vi "Set Color.vi"(9 "index":i32, 10 "Flat Legend":cluster{"Color Box":u32, "String":string}[](array[cluster]), 11 "list in":T1[](array[typedef]) {"Creation Date" format="%<%x>T"; "Last Updated" format="%<%x>T"}) -> (3 "list out":T1[](array[typedef]) {"Creation Date" format="%<%x>T"; "Last Updated" format="%<%x>T"})   [LabVIEW 2018]
uses:
  Type Defs/SR Cluster.ctl
  Type Defs/SR Status.ctl
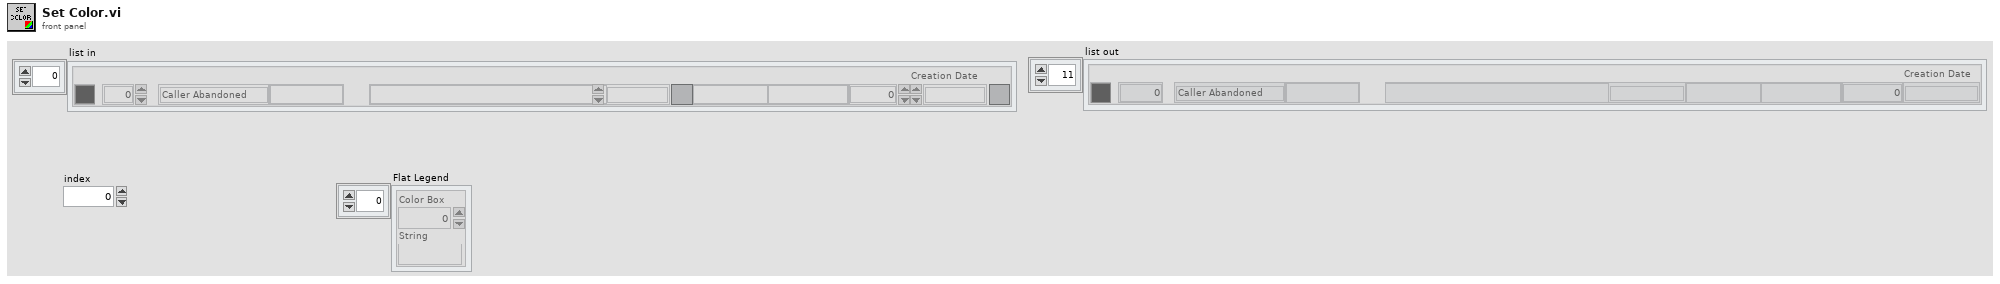
[diagram p1: front panel]
types:
  T1 = typedef "SR Cluster.ctl" = cluster{"Color":u32, "SR Number":i32, "SR Status":T2, "Name":string, "Summary":string, "Last Updated":timestamp, "SR Type":string, "Service Level":string, "Days Open":dbl, "Creation Date":timestamp}
  T2 = typedef "SR Status.ctl" = enum16{"Caller Abandoned", "Created in Error", "Expired", "Forum Resolved AE", "Forum Resolved Customer", "IN WORK", "IN WORK Collab with AES", "IN WORK Collab with PSE", "IN WORK Collab with SE", "IN WORK Customer Added Note", "IN WORK Escalation", "IN WORK Wait on Customer", "Open", "Potentially Resolved", "Presumed Resolved", "RMA Approved for Return", "Resolved", "Passed Off"}
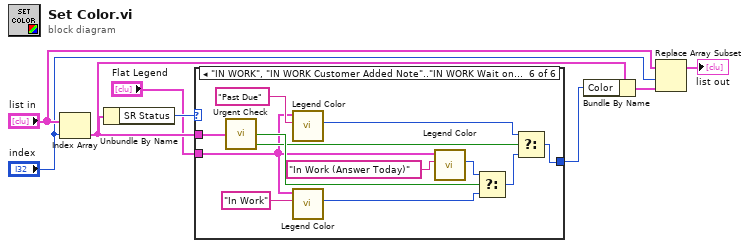
[diagram p0: block diagram]
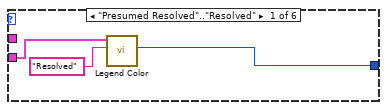
[diagram p2: hidden frame]
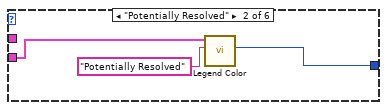
[diagram p3: hidden frame]
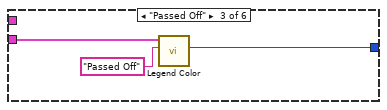
[diagram p4: hidden frame]
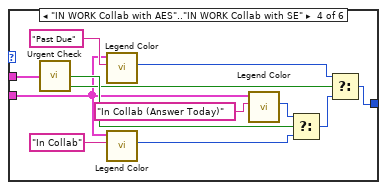
[diagram p5: hidden frame]
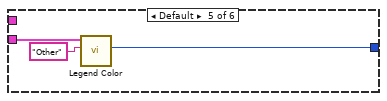
[diagram p6: hidden frame]
diagram:
  n1 = Index Array(array="list in", index="index") -> (element=w2:T1)
  n2 = Unbundle By Name(w2) -> ("SR Status"=w3:T2)
  n3 = case shown="\"IN WORK\", \"IN WORK Customer Added Note\"..\"IN WORK Wait on Customer\"" w3 {
    tunnel: [w10 w13 w16 w20 w30 w33] -> w6
    tunnel: w2 -> [_ _ _ w19 _ w44]
    tunnel: "Flat Legend" -> [w9 w12 w15 w18 w31 w37]
    frame "Presumed Resolved".."Resolved" {
      n4 = call "Legend Color.vi"("label in"="Resolved", "Flat Legend"=w9) -> ("color out"=w10:u32)  [unwired: 9 in]
    }
    frame "Potentially Resolved" {
      n5 = call "Legend Color.vi"("label in"="Potentially Resolved", "Flat Legend"=w12) -> ("color out"=w13:u32)  [unwired: 9 in]
    }
    frame "Passed Off" {
      n6 = call "Legend Color.vi"("label in"="Passed Off", "Flat Legend"=w15) -> ("color out"=w16:u32)  [unwired: 9 in]
    }
    frame "IN WORK Collab with AES".."IN WORK Collab with SE" {
      n7 = call "Urgent Check.vi"("SR Cluster"=w19) -> ("Passed Due?"=w28:bool, "Answer Today?"=w29:bool)  [unwired: 3 in]
      n8 = call "Legend Color.vi"("label in"="Past Due", "Flat Legend"=w18) -> ("color out"=w24:u32)  [unwired: 9 in]
      n9 = call "Legend Color.vi"("label in"="In Collab", "Flat Legend"=w18) -> ("color out"=w26:u32)  [unwired: 9 in]
      n10 = call "Legend Color.vi"("label in"="In Collab (Answer Today)", "Flat Legend"=w18) -> ("color out"=w25:u32)  [unwired: 9 in]
      n11 = Select(t=w25, s=w29, f=w26) -> (s? t:f=w27:u32)
      n12 = Select(t=w24, s=w28, f=w27) -> (s? t:f=w20:u32)
    }
    frame Default {
      n13 = call "Legend Color.vi"("label in"="Other", "Flat Legend"=w31) -> ("color out"=w30:u32)  [unwired: 9 in]
    }
    frame "IN WORK", "IN WORK Customer Added Note".."IN WORK Wait on Customer" {
      n14 = call "Urgent Check.vi"("SR Cluster"=w44) -> ("Passed Due?"=w40:bool, "Answer Today?"=w41:bool)  [unwired: 3 in]
      n15 = call "Legend Color.vi"("label in"="Past Due", "Flat Legend"=w37) -> ("color out"=w34:u32)  [unwired: 9 in]
      n16 = call "Legend Color.vi"("label in"="In Work", "Flat Legend"=w37) -> ("color out"=w36:u32)  [unwired: 9 in]
      n17 = call "Legend Color.vi"("label in"="In Work (Answer Today)", "Flat Legend"=w37) -> ("color out"=w35:u32)  [unwired: 9 in]
      n18 = Select(t=w35, s=w41, f=w36) -> (s? t:f=w39:u32)
      n19 = Select(t=w34, s=w40, f=w39) -> (s? t:f=w33:u32)
    }
  }
  n20 = Bundle By Name(cluster=w2, "Color"=w6) -> (w8:T1)
  n21 = Replace Array Subset(array="list in", new element=w8, index="index") -> (→"list out":T1[])
